vi "Speed Logging-Write data to file.vi"(7 "New file":bool, 8 "error in (no error)":errorcluster, 9 "Speed window data":T1, 10 "Timestamp at trial start":timestamp, 11 "Byte Stream File in":refnum<file>) -> (0 "error out":errorcluster, 2 "Timestamp at trial start":timestamp, 3 "Byte Stream File out":refnum<file>)   [LabVIEW 2020]
uses:
  Typedefs/Speed window notifier data.ctl
  Typedefs/Speed logging states enum.ctl
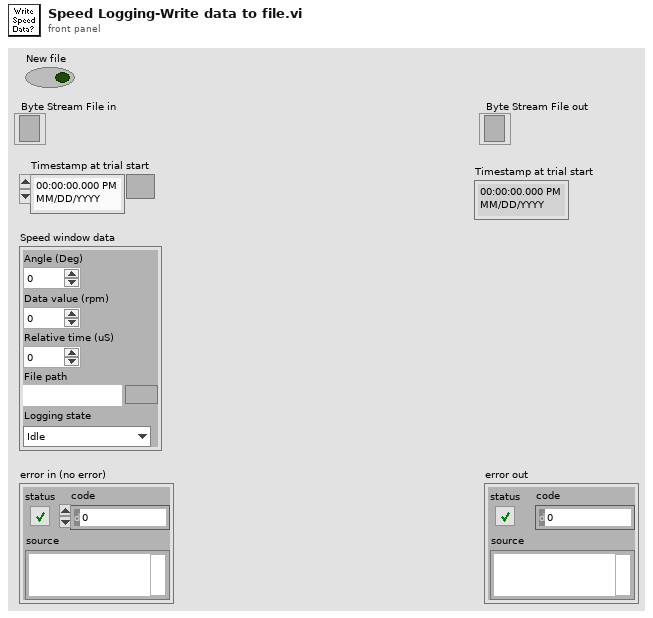
[diagram p1: front panel]
types:
  T1 = typedef "Speed window notifier data.ctl" = cluster{"Angle (Deg)":dbl, "Data value (rpm)":dbl, "Relative time (uS)":i32, "File path":path, "Logging state":T2}
  T2 = typedef "Speed logging states enum.ctl" = enum16{"Idle", "Open file", "Log", "Close file"}
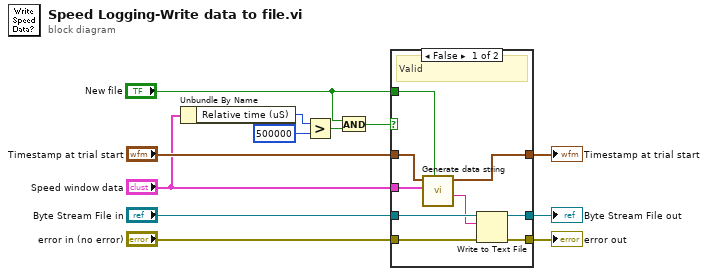
[diagram p0: block diagram]
diagram:
  n1 = Unbundle By Name("Speed window data") -> ("Relative time (uS)"=w6:i32)
  n2 = Greater?(x=w6, y=500000) -> (0:w4:bool)
  n3 = And(x="New file", y=w4) -> (x .and. y?=w3:bool)
  n4 = case shown="False" w3 {
    tunnel: "Timestamp at trial start" -> [w21 w22]
    tunnel: "error in (no error)" -> [w20 w23]
    tunnel: [w19 w23] -> w10
    tunnel: "Byte Stream File in" -> [w18 w24]
    tunnel: [w17 w24] -> w8
    tunnel: "Speed window data" -> [w16 _]
    tunnel: [w14 w22] -> w2
    tunnel: "New file" -> [w13 _]
    frame False {
      # "Valid"
      n5 = call "Generate data string.vi"("New file"=w13, "Speed window data"=w16, "Timestamp at trial start"=w21) -> ("Data String"=w15:string, "Timestamp at trial start"=w14:timestamp)  [unwired: 7 in]
      n6 = Write to Text File(file (use dialog)=w18, text=w15, error in=w20) -> (refnum out=w17:refnum<file>, error out=w19:errorcluster)  [unwired: 1 in, 1 out]
    }
    frame True {
      # "Ignored"
    }
  }
  "error out" <- w10
  "Byte Stream File out" <- w8
  "Timestamp at trial start" <- w2
